vi "open.vi"(8 "error in (no error)":errorcluster caption="错误输入（无错误）", 11 "WebDAV client 输入":refnum<class "WebDAV client.lvclass">) -> (0 "error out":errorcluster caption="错误输出", 3 "WebDAV client 输出":refnum<class "WebDAV client.lvclass">)   [LabVIEW 2016, in "数据传输系统.lvlib" / "update.lvlib" / "WebDAV client.lvclass"]
uses:
  WebDAV client.lvclass
  WebDAV client.lvclass/WebDAV client.ctl
  <vilib>/WebDAVClient/NI_WebDAV.lvlib
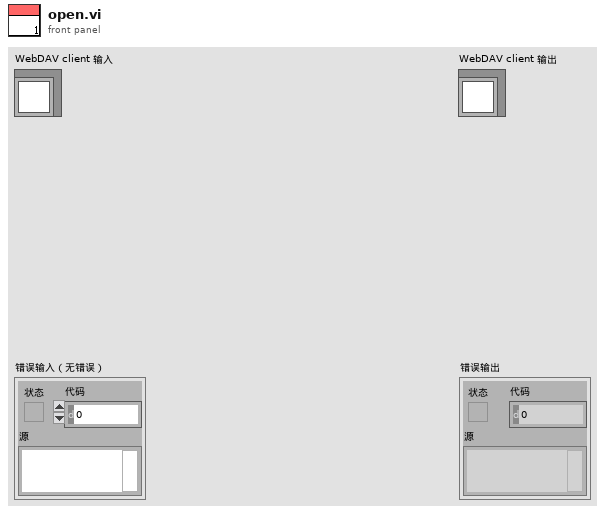
[diagram p1: front panel]
types:
  T1 = cluster{"URL":string, "USER":string, "PASSWORD":string}
  T2 = typedef "NI_WebDAV.lvlib/Asynchronous Session Handle.ctl" = refnum<k1>
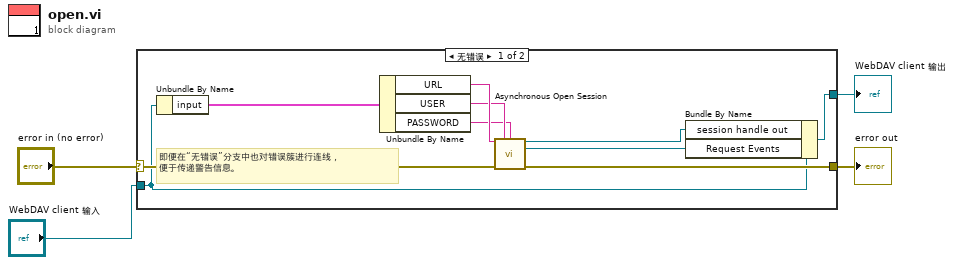
[diagram p0: block diagram]
diagram:
  n1 = case shown="无错误" "error in (no error)" {
    selector: "error in (no error)" -> [w11 w16]
    tunnel: [w10 w16] -> w3
    tunnel: [w8 w15] -> w1
    tunnel: "WebDAV client 输入" -> [w6 w15]
    frame No Error {
      # "即便在“无错误”分支中也对错误簇进行连线，\n便于传递警告信息。"
      n2 = Unbundle By Name(w6) -> ("input"=w5:T1)
      n3 = Unbundle By Name(w5) -> ("URL"=w14:string, "USER"=w13:string, "PASSWORD"=w12:string)
      n4 = call <vilib>:"Asynchronous Open Session.vi"("host uri prefix"=w14, "username"=w13, "password"=w12, "error in (no error)"=w11) -> ("session handle out"=w9:T2, "Request Events"=w7:refnum<event-registration>, "error out"=w10:errorcluster)  [unwired: 9 in]
      n5 = Bundle By Name(cluster=w6, "session handle out"=w9, "Request Events"=w7) -> (w8:refnum<class "WebDAV client.lvclass">)
    }
    frame Error {
    }
  }
  "error out" <- w3
  "WebDAV client 输出" <- w1
